vi "x-element subset.vi"(1 "input array":dbl[](array[numeric]), 2 "x elements":i32) -> (0 "array subset":dbl[](array[numeric]))   [LabVIEW 2023]
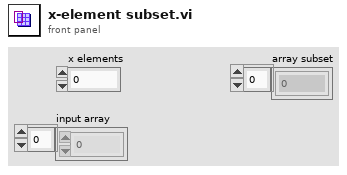
[diagram p1: front panel]
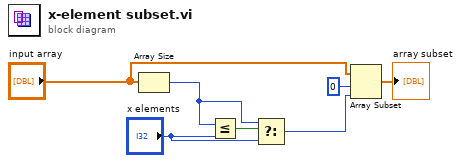
[diagram p0: block diagram]
diagram:
  n1 = Array Size(array="input array") -> (size(s)=w1:i32)
  n2 = Less Or Equal?(x=w1, y="x elements") -> (x <= y?=w3:bool)
  n3 = Select(t=w1, s=w3, f="x elements") -> (s? t:f=w4:i32)
  n4 = Array Subset(array="input array", index=0, length=w4) -> (→"array subset":dbl[])
